vi "Initialize.vi"(11 "pcap Parse and Build in":refnum<class "pcap Parse and Build.lvclass">) -> (3 "pcap Parse and Build out":refnum<class "pcap Parse and Build.lvclass">)   [LabVIEW 2021, in "pcap Parse and Build.lvclass"]
uses:
  pcap Parse and Build.lvclass
  Typedef/Time Format.ctl
  pcap Parse and Build.lvclass/pcap Parse and Build.ctl
  <vilib>/CIF Foundation/CIF Utilities/DataTypes/DataTypes_CIF_U.lvlib
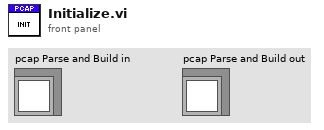
[diagram p1: front panel]
types:
  T1 = typedef "pcap Parse and Build.lvclass/Time Format.ctl" = enum16{"us", "ns"}
  T2 = typedef "DataTypes_CIF_U.lvlib/Endian.ctl" = enum16{"Little Endian", "Big Endian"}
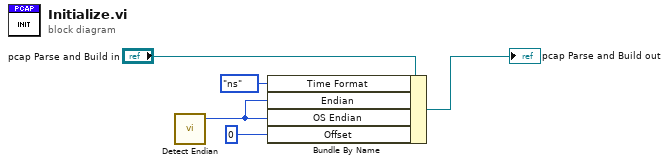
[diagram p0: block diagram]
diagram:
  n1 = call <vilib>:"Detect Endian.vi"() -> ("Endian"=w2:T2)  [unwired: 5 in]
  n2 = Bundle By Name(cluster="pcap Parse and Build in", "Time Format"=Time_Format."ns" ("pcap format.Time Format"), "Endian"=w2, "OS Endian"=w2, "Offset"=0) -> (→"pcap Parse and Build out":refnum<class "pcap Parse and Build.lvclass">)
